vi "create tls dataset.vi"(8 "error in":errorcluster, 11 "lvlibretls server listener":refnum<class "lvlibretls server listener.lvclass">) -> (0 "error out":errorcluster, 3 "TLS HTTP handler dataset out":refnum<class "TLS HTTP handler dataset.lvclass">)   [LabVIEW 2016, in "TLS HTTP handler dataset.lvclass"]
uses:
  TLS HTTP handler dataset.lvclass
  lvlibtls/server/lvlibretls server listener.lvclass
  TLS HTTP handler dataset.lvclass/TLS HTTP handler dataset.ctl
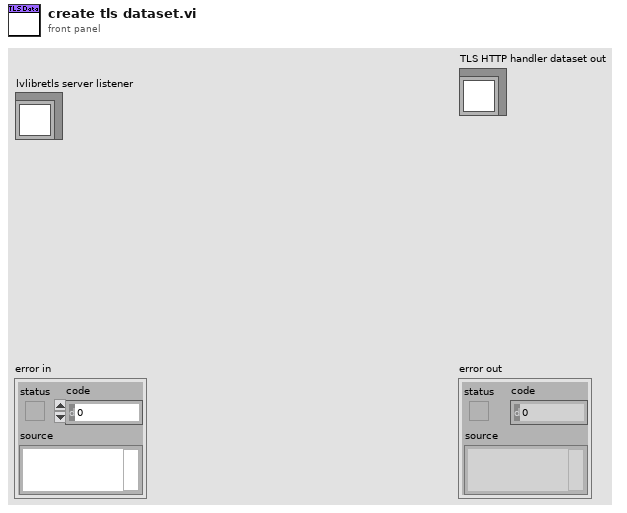
[diagram p1: front panel]
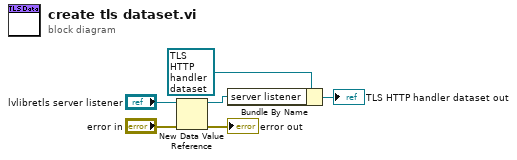
[diagram p0: block diagram]
diagram:
  n1 = New Data Value Reference(data value="lvlibretls server listener", error in="error in") -> (data value reference=w1:refnum<data-value>, error out=→"error out":errorcluster)
  n2 = Bundle By Name(cluster=refnum<class "TLS HTTP handler dataset.lvclass"> refnum ("TLS HTTP handler dataset in"), "server listener"=w1) -> (→"TLS HTTP handler dataset out":refnum<class "TLS HTTP handler dataset.lvclass">)
